vi "Create a test.vi"() -> ()   [LabVIEW 2019]
uses:
  Unit Test Engine Tools.lvlib
  ebda9e4b-04d7-4516-a688-59c92300d774.vi
panel:
  out "error out":errorcluster
  in  "error in (no error)":errorcluster
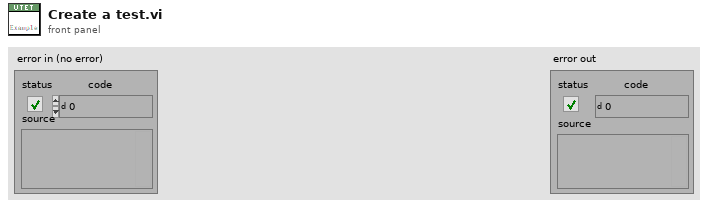
[diagram p1: front panel]
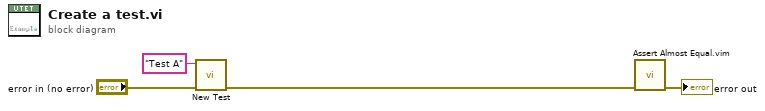
[diagram p0: block diagram]
diagram:
  n1 = call "New Test.vi"("error in (no error)"="error in (no error)", "Test"="Test A") -> ("error out"=w4:errorcluster)  [unwired: 9 in]
  n2 = call "Assert Almost Equal.vim"("error in (no error)"=w4) -> ("error out"=→"error out":errorcluster)  [unwired: 10 in]
